vi "solar Voyager Launch Single Target.vi"(8 "error in (no error)":errorcluster, 9 "Is Main? (F)":bool, 10 "Target Name":string, 11 "solar in":refnum<class "solar.lvclass">) -> (0 "error out":errorcluster, 3 "solar out":refnum<class "solar.lvclass">)   [LabVIEW 2018]
doc: "This launches the Voyager interface for a single target. If the Voyager key is not found in the configuration file, the default configuration is a single TCP Server on port 59200 for each target. Voyager has four configurations:\n- SERVER - TCP server that handles commands and telemetry\n- CLIENT - TCP client that handles commands and telemetry (IP address required)\n- SERVER_CMD - TCP server that only handles incoming commands\n- SERVER_TLM - TCP server that only handles outgoing telemetry"
uses:
  voyager/solar_voy_ctl Port Setup.ctl
  voyager/solar_voy_ctl Port.ctl
  solar.lvclass
  cfg/solar_cfg Read File (Str).vi
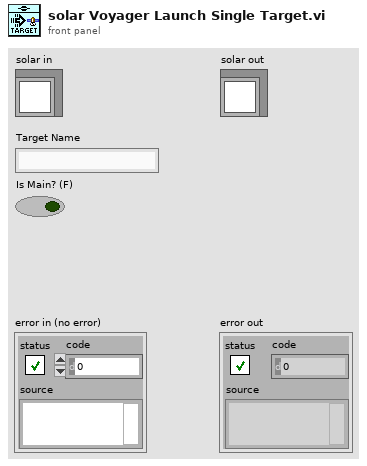
[diagram p1: front panel]
types:
  T1 = typedef "solar_voy_ctl Voyager Refnum.ctl" = refnum<k1>
  T2 = typedef "solar_voy_ctl Port Setup.ctl" = enum8{"SERVER", "CLIENT", "SERVER_CMD", "SERVER_TLM"}
  T3 = typedef "solar_voy_ctl Port.ctl" = cluster{"Setup":T2, "Port":u16, "ServerIP":string, "Target":string}
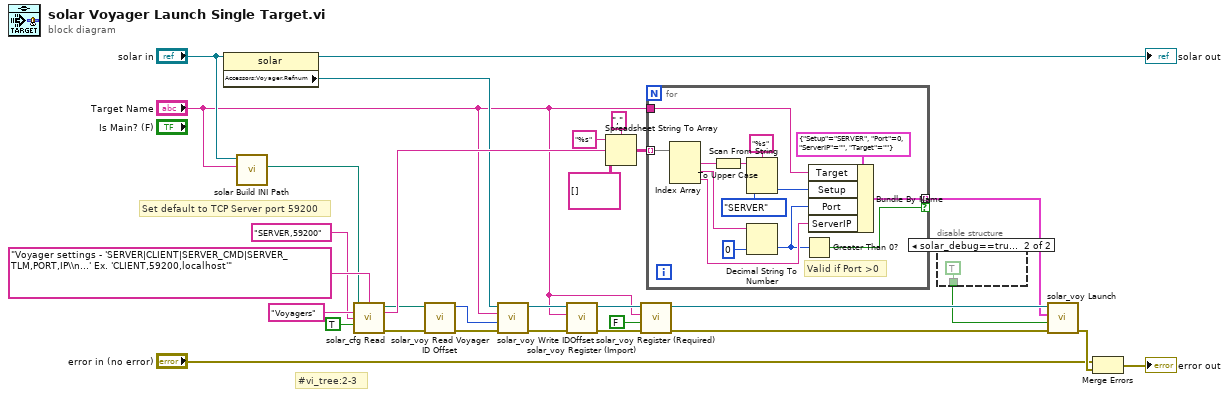
[diagram p0: block diagram]
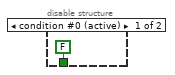
[diagram p2: hidden frame]
diagram:
  # "#vi_tree:2-3"
  # "Set default to TCP Server port 59200"
  n1 = property class="solar"(reference="solar in") -> (reference out=→"solar out":refnum<class "solar.lvclass">, "Accessors:Voyager.Refnum"=w3:T1)  [unwired: 1 in, 1 out]
  n2 = call "solar Build INI Path.vi"("Name"="Target Name", "solar in"="solar in") -> ("appended path"=w9:path)  [unwired: 8 in, 1 out]
  n3 = call-poly "solar_cfg Read.vi"("Config Path (*.ini)"=w9, "Comment"="Voyager settings - 'SERVER|CLIENT|SERVER_CMD|SERVER_TLM,PORT,IP\\n...' Ex. 'CLIENT,59200,localhost'", "Key"="Voyagers", "Value in"="SERVER,59200", "Add Quotes? (T)"=TRUE) -> ("Config Path out"=w4:path, "Value out"=w15:string, "error out"=w6:errorcluster)  [unwired: 7 in, 1 out]
  n4 = call "solar_voy Read Voyager ID Offset.vi"("error in (no error)"=w6, "Config Path in"=w4) -> ("error out"=w8:errorcluster, "VoyagerIDOffset"=w7:u16)  [unwired: 8 in]
  n5 = call "solar_voy Write IDOffset.vi"("error in (no error)"=w8, "ID Offset"=w7, "Target Name"="Target Name", "Voyager Refnum in"=w3) -> ("error out"=w5:errorcluster, "Voyager Refnum out"=w2:T1)  [unwired: 6 in]
  n6 = call "solar_voy Register (Import).vi"("error in (no error)"=w5, "Target Name"="Target Name", "Voyager Refnum in"=w2) -> ("error out"=w28:errorcluster, "Voyager Refnum out"=w27:T1)  [unwired: 7 in]
  n7 = Spreadsheet String To Array(delimiter (Tab)=",", format string="%s", spreadsheet string=w15, array type (2D Dbl)=string[][] []) -> (array=w19:string[][])
  n8 = call "solar_voy Register (Required).vi"("error in (no error)"=w28, "Override If Exists? (F)"=FALSE, "Target Name"="Target Name", "Voyager Refnum in"=w27) -> ("error out"=w26:errorcluster, "Voyager Refnum out"=w25:T1)  [unwired: 6 in]
  n9 = for {
    tunnel: w19 -> [w44] mode=indexing
    tunnel: [w38] -> w13 mode=indexing if=w37
    tunnel: "Target Name" -> [w31]
    # "Valid if Port >0"
    n10 = Index Array(array=w44) -> (element #1=w36:string, element #2=w43:string, element #3=w40:string)  [unwired: 3 in]
    n11 = To Upper Case(1:w36) -> (0:w34:string)
    n12 = Scan From String(format string="%s", input string=w34, default 1=solar_voy_ctl_Port_Setup."SERVER" ("Setup")) -> (output 1=w32:T2)  [unwired: 2 in, 3 out]
    n13 = Decimal String To Number(string=w43, default (0L)=u16 0 ("Port")) -> (number=w39:u16)  [unwired: 1 in, 1 out]
    n14 = Greater Than 0?(x=w39) -> (x > 0?=w37:bool)
    n15 = Bundle By Name(cluster=T3 {"Setup"=enum."SERVER", "Port"=0, "ServerIP"="", "Target"=""} ("Port"), "Target"=w31, "Setup"=w32, "Port"=w39, "ServerIP"=w40) -> (w38:T3)
  }
  n16 = disable-structure shown="solar_debug==true" {
    disable-tunnel: [FALSE TRUE ("Open FP? (F)")] -> w11
    frame condition #0 (active) {
    }
    frame condition #1 {
    }
  }
  n17 = call "solar_voy Launch.vi"("error in (no error)"=w26, "Open FP? (F)"=w11, "Ports"=w13, "Voyager Refnum in"=w25) -> ("error out"=w29:errorcluster)  [unwired: 6 in, 1 out]
  n18 = Merge Errors("error in (no error)", w29) -> (→"error out":errorcluster)
